vi "SineMoveDynamic.vi"(6 "frequency2":dbl=3.0 format="%#_13g", 7 "frequency1":dbl=3.0 format="%#_13g", 8 "error in (no error)":errorcluster caption="错误输入（无错误）", 9 "limit":dbl=40.0 format="%#_13g", 11 "RandomMoveBool 输入":refnum<class "RandomMoveBool.lvclass">) -> (0 "error out":errorcluster caption="错误输出", 3 "RandomMoveBool 输出":refnum<class "RandomMoveBool.lvclass">)   [LabVIEW 2018, in "RandomMoveBool.lvclass"]
uses:
  RandomMoveBool.lvclass
  <vilib>/Utility/miscctls.llb/LVPositionTypeDef.ctl
  RandomMoveBool.lvclass/RandomMoveBool.ctl
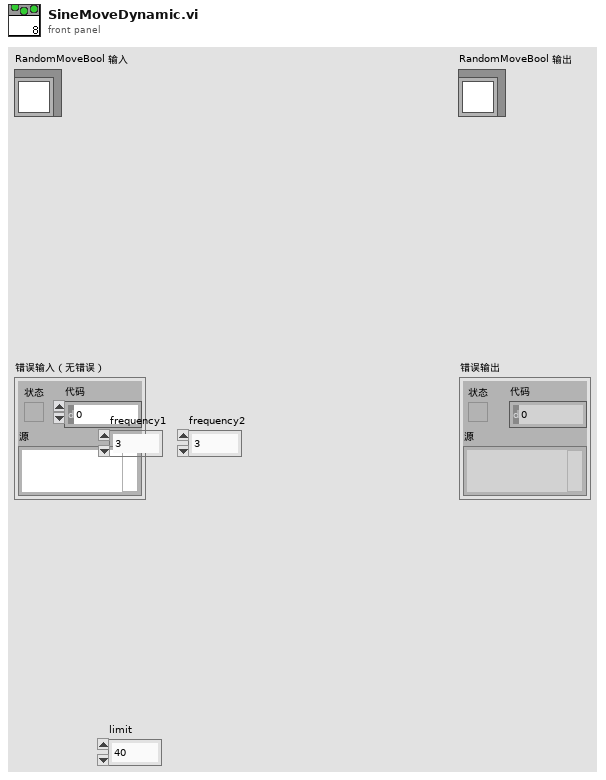
[diagram p1: front panel]
types:
  T1 = typedef "LVPositionTypeDef.ctl" = cluster{"Left":i32, "Top":i32}
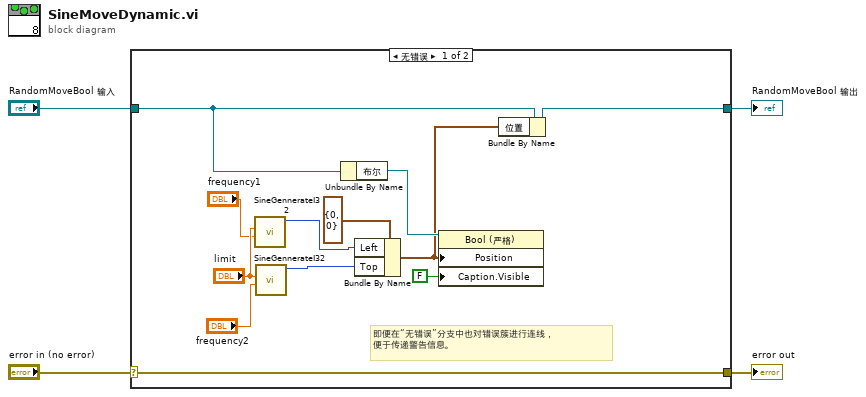
[diagram p0: block diagram]
diagram:
  n1 = case shown="无错误" "error in (no error)" {
    selector: "error in (no error)" -> [w16 w18]
    tunnel: [w16 w18] -> w3
    tunnel: [w6 w17] -> w1
    tunnel: "RandomMoveBool 输入" -> [w7 w17]
    frame No Error {
      # "即便在“无错误”分支中也对错误簇进行连线，\n便于传递警告信息。"
      n2 = call "SineGennerateI32.vi"("frequency"="frequency1", "limit"="limit") -> ("y"=w11:i32)  [unwired: 8 in, 1 out]
      n3 = call "SineGennerateI32.vi"("frequency"="frequency2", "limit"="limit") -> ("y"=w12:i32)  [unwired: 8 in, 1 out]
      n4 = Unbundle By Name(w7) -> ("布尔"=w15:refnum<vi>)
      n5 = Bundle By Name(cluster=T1 {"Left"=0, "Top"=0} ("位置"), "Left"=w11, "Top"=w12) -> (w5:T1)
      n6 = property class="Bool (严格)"(reference=w15, "Position"=w5, "Caption.Visible"=FALSE ("标题.可见")) -> ()  [unwired: 1 in, 2 out]
      n7 = Bundle By Name(cluster=w7, "位置"=w5) -> (w6:refnum<class "RandomMoveBool.lvclass">)
    }
    frame Error {
    }
  }
  "error out" <- w3
  "RandomMoveBool 输出" <- w1
